vi "OLED显示实验.vi"() -> ()   [LabVIEW 2011]
uses:
  <vilib>/STM32_DriverVI_Interface_F4/OLED/OLED_Clear_Mode_F4.ctl
  <vilib>/STM32_DriverVI_Interface_F4/OLED/OLED_Fill_Mode_F4.ctl
  <vilib>/STM32_DriverVI_Interface_F4/LCD/Font_Size_F4.ctl
  <vilib>/STM32_DriverVI_Interface_F4/OLED/OLED_Show_Mode_F4.ctl
  <vilib>/STM32_DriverVI_Interface_F4/OLED/OLED_Comm_Mode_F4.ctl
  <vilib>/STM32_DriverVI_Interface_F4/OLED/OLED Init_F4.vi
  <vilib>/STM32_DriverVI_Interface_F4/OLED/OLED Fill Rectangle_F4.vi
  <vilib>/STM32_DriverVI_Interface_F4/OLED/OLED Show String_F4.vi
  <vilib>/STM32_DriverVI_Interface_F4/OLED/OLED Clear Screen_F4.vi
panel:
  in  "OLED_Show_Mode":T1=enum."正常显示"
  in  "Font_Size":T2=enum."Big_Font（16）"
  in  "Y_Position":u16 max=320
  in  "X_Position":u16 max=320
  in  "Y2_Position":u16 max=320
  in  "X2_Position":u16 max=320
  in  "OLED_Fill_Mode":T3=enum."填充"
  in  "Y1_Position":u16 max=320
  in  "X1_Position":u16 max=320
  in  "OLED_Clear_Mode":T4
  in  "停止":bool
  out "正在运行":i32
  in  "Fill":bool
  in  "Show":bool
  in  "Clear":bool
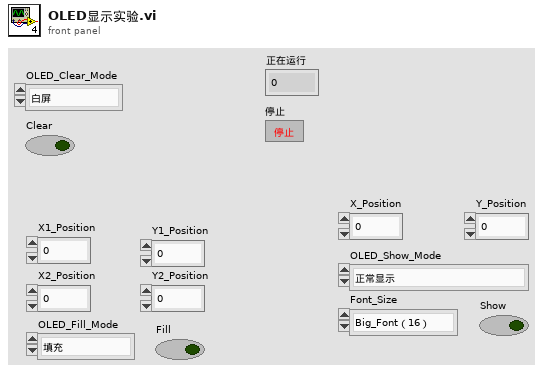
[diagram p1: front panel]
types:
  T1 = typedef "OLED_Show_Mode_F4.ctl" = enum8{"反白显示", "正常显示"}
  T2 = typedef "Font_Size_F4.ctl" = enum8{"Small_Font（12）", "Big_Font（16）"}
  T3 = typedef "OLED_Fill_Mode_F4.ctl" = enum8{"清空", "填充"}
  T4 = typedef "OLED_Clear_Mode_F4.ctl" = enum8{"白屏", "黑屏"}
  T5 = typedef "OLED_Comm_Mode_F4.ctl" = enum8{"4线制SPI通信", "8080并口通信"}
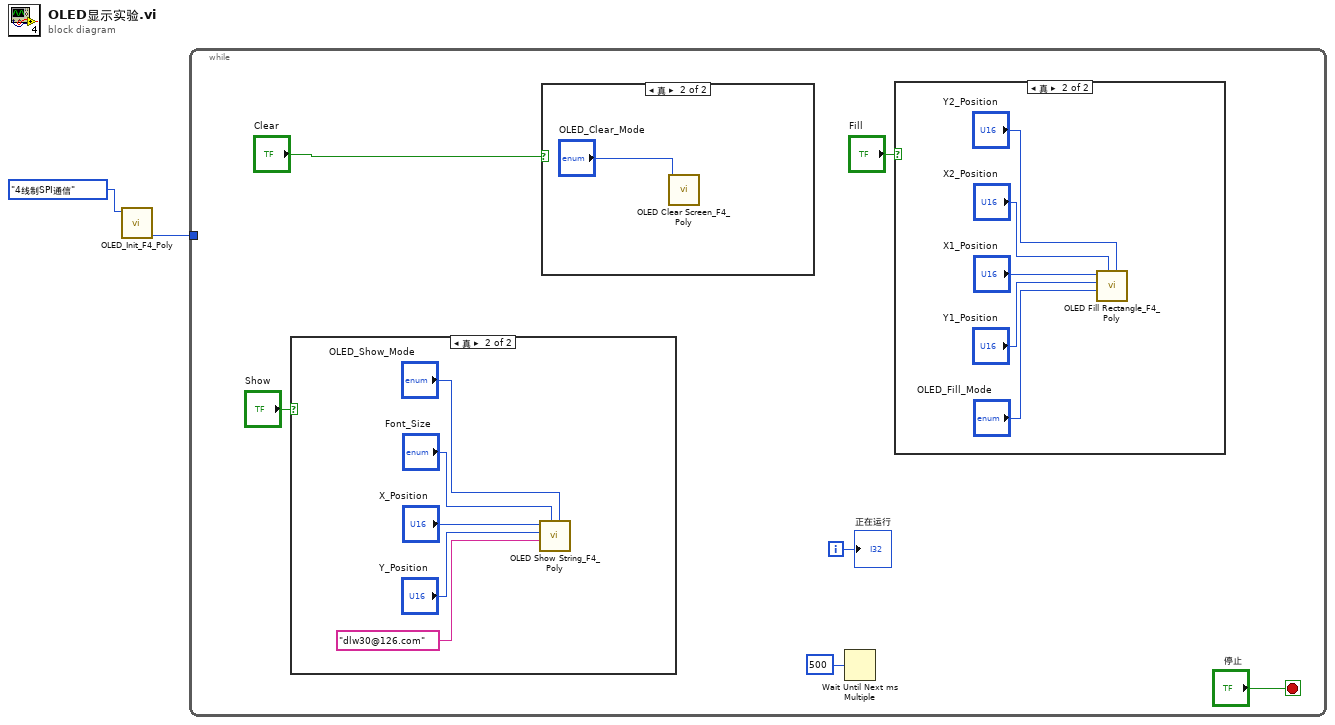
[diagram p0: block diagram]
diagram:
  n1 = call-poly <vilib>:"OLED_Init_F4_Poly.vi"("OLED_Line_Mode"=OLED_Comm_Mode_F4."4线制SPI通信") -> ("err_out"=w1:u8)  [unwired: 10 in]
  n2 = while {
    tunnel: w1 -> [_]
    i -> [w5]
    stop <- "停止" stop-if-true
    n3 = case shown="真" "Show" {
      frame False {
      }
      frame True {
        n4 = call-poly <vilib>:"OLED Show String_F4_Poly.vi"("OLED_Show_Mode"="OLED_Show_Mode", "Font_Size"="Font_Size", "String"="dlw30@126.com", "Y_Position"="Y_Position", "X_Position"="X_Position") -> ()  [unwired: 6 in, 1 out]
      }
    }
    n5 = case shown="真" "Clear" {
      frame False {
      }
      frame True {
        n6 = call-poly <vilib>:"OLED Clear Screen_F4_Poly.vi"("OLED_Clear_Mode"="OLED_Clear_Mode") -> ()  [unwired: 10 in, 1 out]
      }
    }
    n7 = Wait Until Next ms Multiple(millisecond multiple=u32 500 ("毫秒倍数")) -> ()  [unwired: 1 out]
    n8 = case shown="真" "Fill" {
      frame False {
      }
      frame True {
        n9 = call-poly <vilib>:"OLED Fill Rectangle_F4_Poly.vi"("Y2_Position"="Y2_Position", "X2_Position"="X2_Position", "OLED_Fill_Mode"="OLED_Fill_Mode", "Y1_Position"="Y1_Position", "X1_Position"="X1_Position") -> ()  [unwired: 6 in, 1 out]
      }
    }
    "正在运行" <- w5
  }
